vi "LCR_Init.vi"(8 "error in (no error)":errorcluster, 11 "LCRControl in":refnum<class "LCRControl.lvclass">) -> (0 "error out":errorcluster, 3 "LCRControl out":refnum<class "LCRControl.lvclass">)   [LabVIEW 2013, in "LCRControl.lvclass"]
uses:
  LCRControl.lvclass
  InstrControl.lvclass
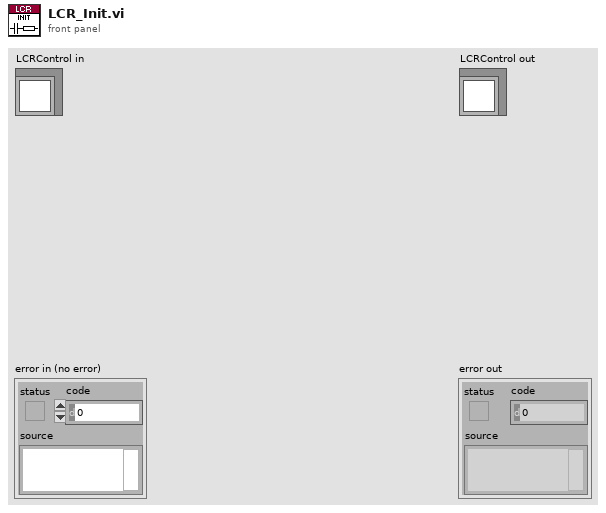
[diagram p1: front panel]
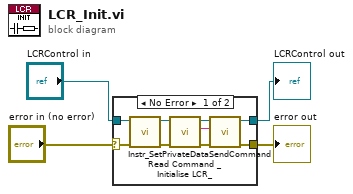
[diagram p0: block diagram]
diagram:
  n1 = case shown="No Error" "error in (no error)" {
    selector: "error in (no error)" -> [w7 w15]
    tunnel: [w9 w15] -> w3
    tunnel: [w13 w14] -> w1
    tunnel: "LCRControl in" -> [w8 w14]
    frame No Error {
      n2 = call-dynamic "Instr_SetPrivateData.vi"("error in (no error)"=w7, "LCRControl in"=w8) -> ("error out"=w5:errorcluster, "LCRControl out"=w6:refnum<class "LCRControl.lvclass">)  [unwired: 8 in]
      n3 = call-dynamic "Read Command _Initialise LCR_.vi"("error in (no error)"=w5, "LCRControl in"=w6) -> ("error out"=w10:errorcluster, "Command \"Initialise LCR\""=w11:string, "LCRControl out"=w12:refnum<class "LCRControl.lvclass">)  [unwired: 7 in]
      n4 = call "SendCommand.vi"("error in (no error)"=w10, "Command string"=w11, "InstControl in"=w12) -> ("error out"=w9:errorcluster, "InstControl out"=w13:refnum<class "LCRControl.lvclass">)  [unwired: 7 in]
    }
    frame Error {
    }
  }
  "error out" <- w3
  "LCRControl out" <- w1
